vi "TauxReussie.vi"(1 "?":bool) -> ()   [LabVIEW 2024]
uses:
  <vilib>/drjdpowell/SQLite Library/SQL Connection/Open (string).vi
  <vilib>/drjdpowell/SQLite Library/SQL Connection/Execute SQL.vi
  <vilib>/drjdpowell/SQLite Library/SQL Connection/Connection.lvclass
  <vilib>/drjdpowell/SQLite Library/SQLite.lvlib
panel:
  # "Taux de réussite de livraison\nSi taux > 0.85 => Réussi\nSinon Echouée"
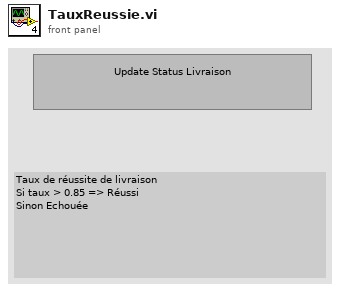
[diagram p1: front panel]
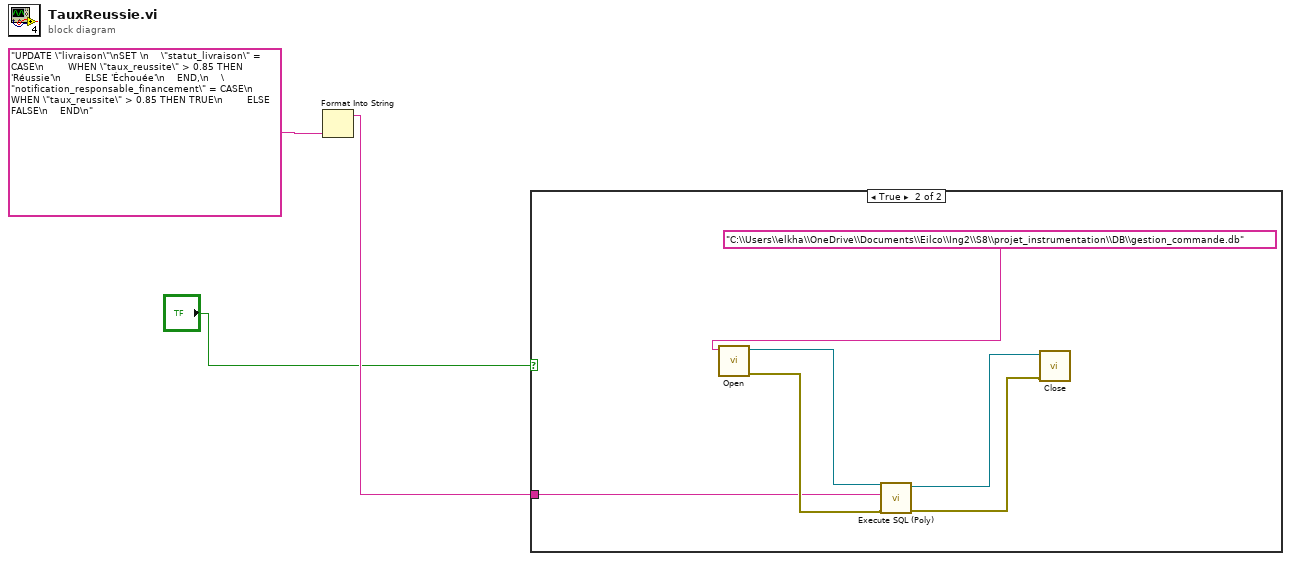
[diagram p0: block diagram]
diagram:
  n1 = Format Into String("UPDATE \"livraison\"\nSET \n    \"statut_livraison\" = CASE\n        WHEN \"taux_reussite\" > 0.85 THEN 'Réussie'\n        ELSE 'Échouée'\n    END,\n    \"notification_responsable_financement\" = CASE\n        WHEN \"taux_reussite\" > 0.85 THEN TRUE\n        ELSE FALSE\n    END\n" ("SQL")) -> (resulting string=w2:string)  [unwired: 3 in, 1 out]
  n2 = case shown="True" "?" {
    tunnel: w2 -> [_ w5]
    frame False {
    }
    frame True {
      n3 = call-poly <vilib>:"Open.vi"("db file"="C:\\Users\\elkha\\OneDrive\\Documents\\Eilco\\Ing2\\S8\\projet_instrumentation\\DB\\gestion_commande.db") -> ("error out"=w9:errorcluster, "SQLite Connection"=w6:refnum<class "Connection.lvclass">)  [unwired: 9 in]
      n4 = call-poly <vilib>:"Execute SQL (Poly).vi"("error in (no error)"=w9, "SQL"=w5, "SQLite Connection in"=w6) -> ("error out"=w8:errorcluster, "SQLite Connection"=w7:refnum<class "Connection.lvclass">)  [unwired: 5 in, 2 out]
      n5 = call-dynamic "Close.vi"("error in (no error)"=w8, "SQLite Connection in"=w7) -> ()  [unwired: 9 in, 1 out]
    }
  }
